vi "Write DATA_Notifier.vi"(8 "error in (no error)":errorcluster, 10 "DATA":T1, 11 "Notifiers in":refnum<class "Notifiers.lvclass">) -> (0 "error out":errorcluster, 3 "Notifiers out":refnum<class "Notifiers.lvclass">)   [LabVIEW 2020, in "Notifiers.lvclass"]
doc: "Data cluster accessors to write the data."
uses:
  Classes/Children/Intra-Application/Children/With Data/Children/Notifiers/Notifiers.lvclass
  Classes/Children/Intra-Application/Children/With Data/Children/Notifiers/Notifiers.lvclass/Notifiers.ctl
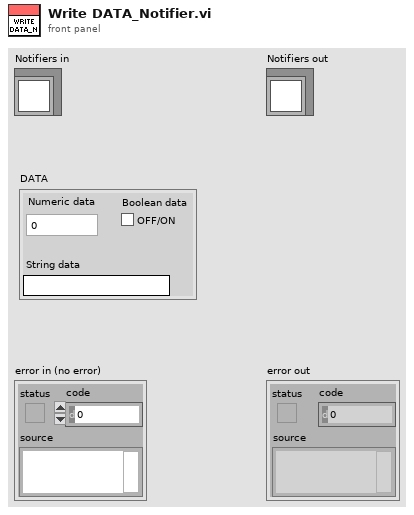
[diagram p1: front panel]
types:
  T1 = cluster{"Numeric data":dbl, "String data":string, "Boolean data":bool}
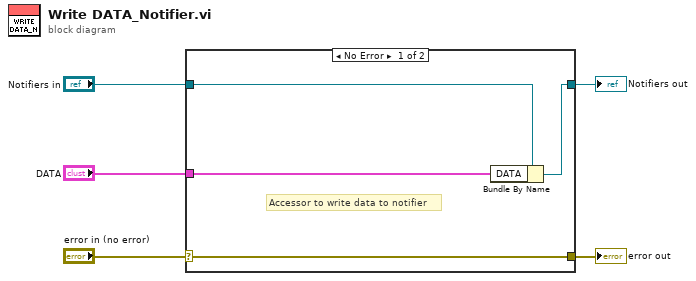
[diagram p0: block diagram]
diagram:
  n1 = case shown="No Error" "error in (no error)" {
    selector: "error in (no error)" -> [w9 w10]
    tunnel: [w9 w10] -> w4
    tunnel: [w7 w11] -> w2
    tunnel: "Notifiers in" -> [w8 w11]
    tunnel: "DATA" -> [w6 _]
    frame No Error {
      # "Accessor to write data to notifier"
      n2 = Bundle By Name(cluster=w8, "DATA"=w6) -> (w7:refnum<class "Notifiers.lvclass">)
    }
    frame Error {
    }
  }
  "error out" <- w4
  "Notifiers out" <- w2
